vi "SendCommand.vi"(6 "error in":errorcluster, 8 "Command":string, 9 "Device Handle":u64) -> (0 "error out":errorcluster, 1 "Number":dbl format="%.2f", 2 "String":string, 3 "Dup Handle":u64)   [LabVIEW 2018, in "Laser.lvlib"]
uses:
  Laser.lvlib
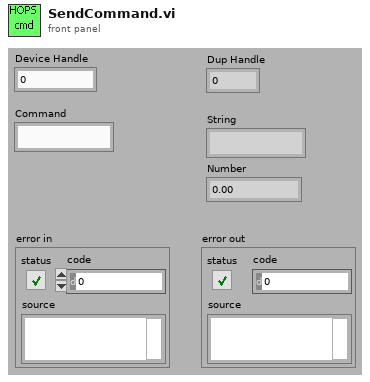
[diagram p1: front panel]
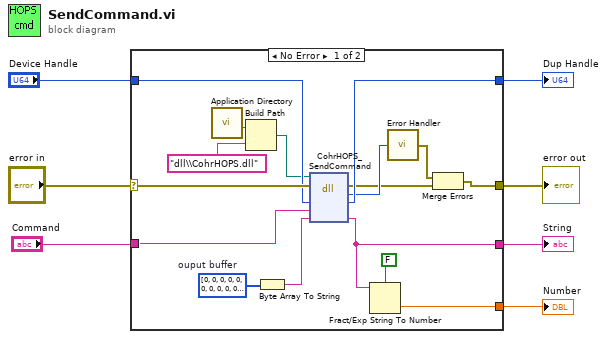
[diagram p0: block diagram]
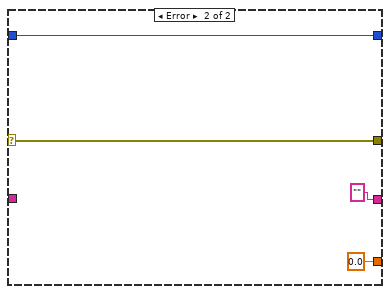
[diagram p2: hidden frame]
diagram:
  n1 = case shown="No Error" "error in" {
    selector: "error in" -> [w20 w27]
    tunnel: "Command" -> [w23 _]
    tunnel: [w17 w27] -> w6
    tunnel: [w21 w26] -> w5
    tunnel: "Device Handle" -> [w19 w26]
    tunnel: [w12 0.0] -> w2
    tunnel: [w11 "" ("arg3")] -> w1
    frame No Error {
      w14 = u8[] [0, 0, 0, 0, 0, 0, 0, 0, 0, 0, 0, 0, 0, 0, 0, 0, 0, 0, 0, 0, 0, 0, 0, 0, 0, 0, 0, 0, 0, 0, 0, 0, 0, 0, 0, 0, 0, 0, 0, 0, 0, 0, 0, 0, 0, 0, 0, 0, 0, 0, 0, 0, 0, 0, 0, 0, 0, 0, 0, 0, 0, 0, 0, 0, 0, 0, 0, 0, 0, 0, 0, 0, 0, 0, 0, 0, 0, 0, 0, 0, 0, 0, 0, 0, 0, 0, 0, 0, 0, 0, 0, 0, 0, 0, 0, 0, 0, 0, 0, 0, 1]  # ouput buffer
      n2 = call <vilib>:"Application Directory.vi"() -> ("Application Directory"=w10:path)
      n3 = Build Path(base path=w10, name or relative path="dll\\CohrHOPS.dll") -> (appended path=w8:path)
      n4 = Byte Array To String(unsigned byte array=w14) -> (string=w13:string)
      n5 = dll-call lib="?" fn="CohrHOPS_SendCommand"(path in=w8, error in=w20, "arg1"=w19, "arg2"=w23, "arg3"=w13) -> (error out=w15:errorcluster, "return type"=w18:i32, "arg1"=w21:u64, "arg3"=w11:string)  [unwired: 2 in, 1 out]
      n6 = Fract/Exp String To Number(use system decimal point (T)=FALSE, string=w11) -> (number=w12:dbl)  [unwired: 2 in, 1 out]
      n7 = call "Error Handler.vi"("Return Value"=w18) -> ("error out"=w16:errorcluster)
      n8 = Merge Errors(w16, w15) -> (w17:errorcluster)
    }
    frame Error {
    }
  }
  "error out" <- w6
  "Dup Handle" <- w5
  "Number" <- w2
  "String" <- w1
